vi "Host_HoppingScan(XY_FPGAWithin).vi"() -> ()   [LabVIEW 2014]
uses:
  <vilib>/userdefined/High Color/nirio_resource_hc.ctl
  <vilib>/Math Plots/3D Math Plots/3D Surface/3D Surface XCtrl/3D Surface.xctl
  <vilib>/FPGAPlugInAG/PCIe-7851R/niLvFpga_Open_PCIe-7851R.vi
  <vilib>/rvi/interface/common/dynamic/niFpgaDynamicAddResources.vi
  <vilib>/Utility/error.llb/Error Cluster From Error Code.vi
  <vilib>/rvi/errors/niLvFpgaAdjustHostInterfaceError.vi
  <vilib>/FPGAPlugInAG/Dynamic/niLvFpga_Run_Dynamic.vi
  <vilib>/FPGAPlugInAG/Dynamic/niLvFpga_Close_Dynamic.vi
  <vilib>/Math Plots/3D Math Plots/3D Surface/3D Surface Datatype/Public/Plot Helper (Matrix).vi
  <vilib>/rvi/interface/nirviOpenFPGA/nirviOpenFPGA.xnode
  FPGA Bitfiles/XZFPGAWithinHopp_FPGATarget_HoppingStepModif_nhH-EM1Hrjw.lvbitx
  <vilib>/rvi/interface/nirviReadWriteControl/nirviReadWriteControl.xnode
  <vilib>/rvi/interface/nirviMethod/nirviMethod.xnode
  <vilib>/rvi/interface/nirviCloseFPGA/nirviCloseFPGA.xnode
  NiFpgaLv.dll
  <vilib>/rvi/interface/Simulation/niFpgaSimulationCallBeginRW.vi
  <vilib>/FPGAPlugInAG/Dynamic/niLvFpga_ReadFifo_Dynamic.vi
  <vilib>/rvi/errors/niLvFpgaMergeErrorWithErrorCode.vi
  <vilib>/Math Plots/3D Math Plots/3D Surface/3D Surface Datatype/3D Surface Datatype.lvclass
panel:
  out "YGets":i32
  out "XGets":u32
  out "ZPos":i16(graph)
  out "3D Surface":refnum<class "3D Plot Datatype.lvclass">[](xcontrol)
  in  "stop":bool
  in  "PIXYZ":T1
  in  "InitZOffset":i32
  in  "MajorWithdraw":i32
  in  "YInitPos um":dbl
  in  "YStepLen um":dbl
  in  "YNum":i32
  in  "XInitPos um":dbl
  in  "XStepLen um":dbl
  in  "XNum":i32
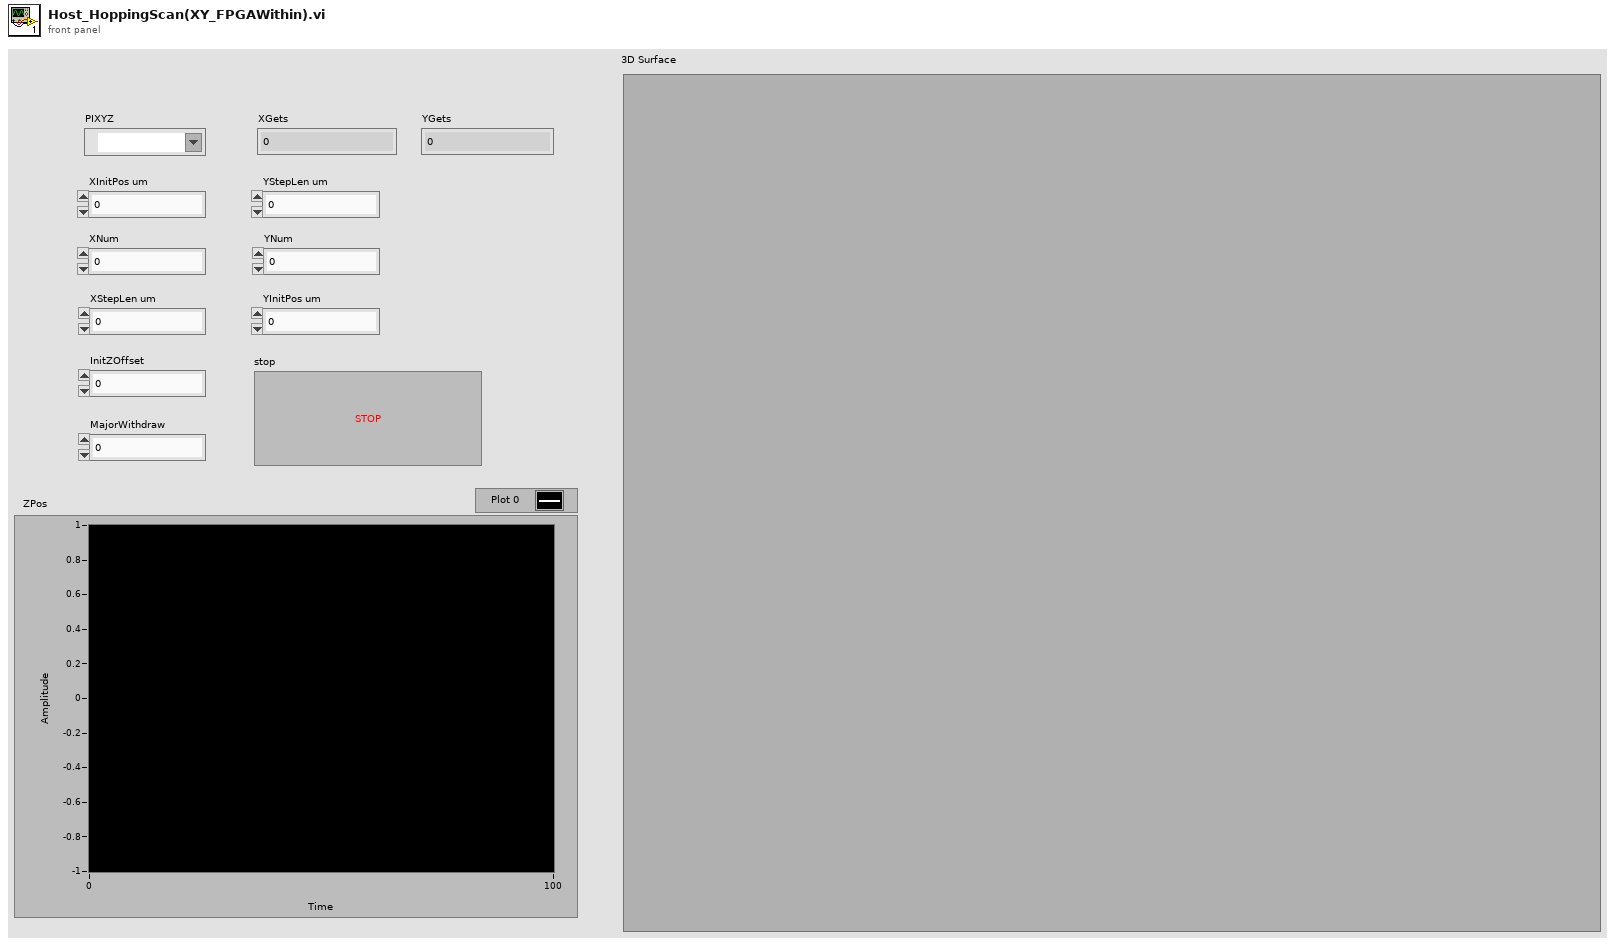
[diagram p1: front panel]
types:
  T1 = typedef "nirio_resource_hc.ctl" = tag
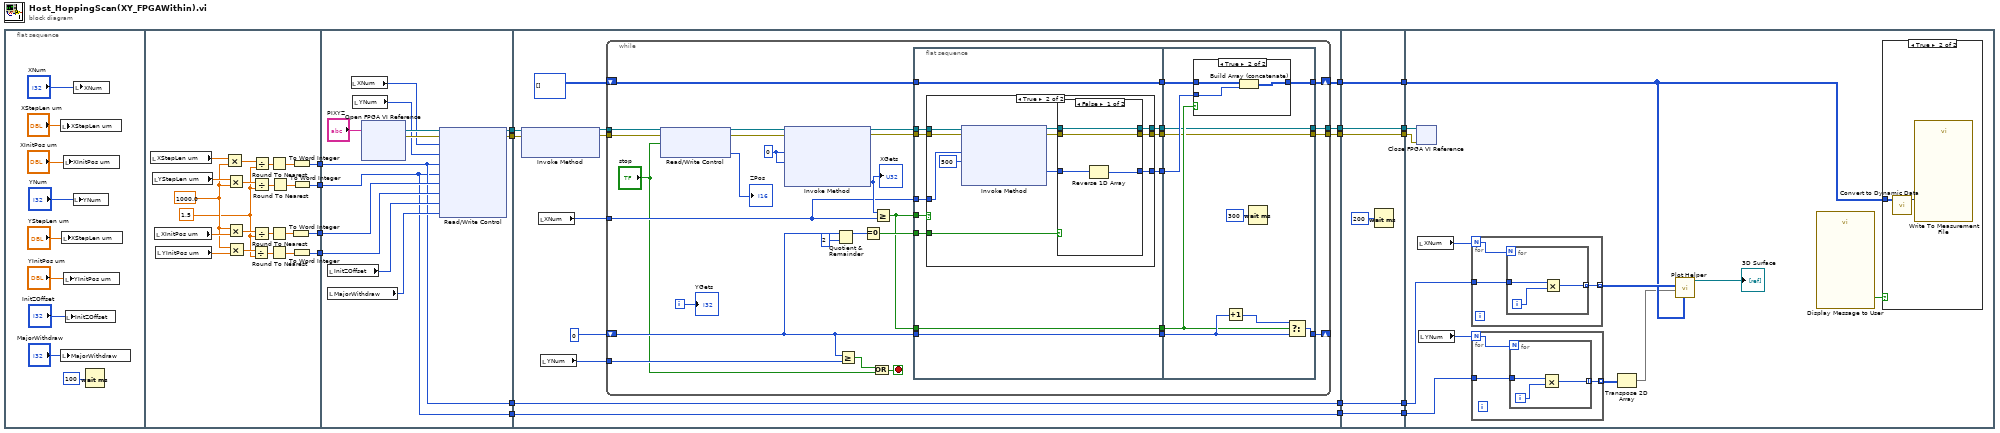
[diagram p0: block diagram]
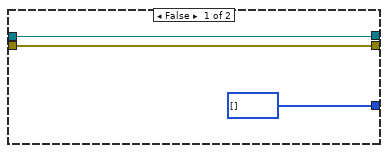
[diagram p2: hidden frame]
diagram:
  n1 = flat-sequence {
    tunnel: [w41] -> w16
    tunnel: [w40] -> w15
    tunnel: [w29] -> w14
    tunnel: [w28] -> w13
    tunnel: [w59] -> w18
    tunnel: [w58] -> w17
    tunnel: w16 -> [w51]
    tunnel: w15 -> [w50]
    tunnel: w14 -> [w55]
    tunnel: w13 -> [w54]
    tunnel: [w51] -> w6
    tunnel: [w50] -> w4
    tunnel: w18 -> [w75]
    tunnel: w17 -> [w74]
    tunnel: [w67] -> w11
    tunnel: [w66] -> w10
    tunnel: [w65] -> w9
    tunnel: w6 -> [w63]
    tunnel: [w64] -> w5
    tunnel: w4 -> [w64]
    tunnel: [w63] -> w3
    tunnel: [w157] -> w12
    tunnel: w11 -> [w157]
    tunnel: w10 -> [w156]
    tunnel: w9 -> [w155]
    tunnel: [w156] -> w8
    tunnel: [w155] -> w7
    tunnel: w5 -> [w153]
    tunnel: w3 -> [w154]
    tunnel: [w154] -> w2
    tunnel: [w153] -> w1
    tunnel: w12 -> [w161]
    tunnel: w8 -> [w170]
    tunnel: w7 -> [w169]
    tunnel: w2 -> [w165]
    tunnel: w1 -> [w164]
    frame #0 {
      n2 = local write "XStepLen um"("XStepLen um") -> ()
      n3 = local write "MajorWithdraw"("MajorWithdraw") -> ()
      n4 = local write "XStepLen um"("YStepLen um") -> ()
      n5 = local write "XInitPos um"("XInitPos um") -> ()
      n6 = local write "YInitPos um"("YInitPos um") -> ()
      n7 = local write "InitZOffset"("InitZOffset") -> ()
      n8 = local write "YNum"("YNum") -> ()
      n9 = local write "XNum"("XNum") -> ()
      n10 = Wait (ms)(milliseconds to wait=u32 100) -> ()  [unwired: 1 out]
    }
    frame #1 {
      w30 = 1.5
      w37 = 1000.0
      n11 = local read "XStepLen um"() -> (w47:dbl)
      n12 = local read "YStepLen um"() -> (w46:dbl)
      n13 = local read "XInitPos um"() -> (w39:dbl)
      n14 = local read "YInitPos um"() -> (w38:dbl)
      n15 = Multiply(x=w47, y=w37) -> (x*y=w48:dbl)
      n16 = Multiply(x=w46, y=w37) -> (x*y=w49:dbl)
      n17 = Multiply(x=w37, y=w39) -> (x*y=w32:dbl)
      n18 = Multiply(x=w37, y=w38) -> (x*y=w31:dbl)
      n19 = Divide(x=w31, y=w30) -> (x/y=w35:dbl)
      n20 = Divide(x=w49, y=w30) -> (x/y=w44:dbl)
      n21 = Divide(x=w32, y=w30) -> (x/y=w36:dbl)
      n22 = Divide(x=w48, y=w30) -> (x/y=w45:dbl)
      n23 = Round To Nearest(number=w36) -> (nearest integer value=w34:dbl)
      n24 = Round To Nearest(number=w45) -> (nearest integer value=w43:dbl)
      n25 = Round To Nearest(number=w35) -> (nearest integer value=w33:dbl)
      n26 = Round To Nearest(number=w44) -> (nearest integer value=w42:dbl)
      n27 = To Word Integer(number=w34) -> (16bit integer=w29:i16)
      n28 = To Word Integer(number=w43) -> (16bit integer=w41:i16)
      n29 = To Word Integer(number=w33) -> (16bit integer=w28:i16)
      n30 = To Word Integer(number=w42) -> (16bit integer=w40:i16)
    }
    frame #2 {
      n31 = local read "InitZOffset"() -> (w53:i32)
      n32 = local read "MajorWithdraw"() -> (w52:i32)
      n33 = local read "XNum"() -> (w57:i32)
      n34 = local read "YNum"() -> (w56:i32)
      n35 = xnode "Open FPGA VI Reference"("resource name"="PIXYZ") -> ("FPGA VI Reference Out"=w61:refnum<k20>, "error out"=w60:errorcluster)  [unwired: 1 in]
      n36 = xnode "Read/Write Control"("FPGA VI Reference In"=w61, "error in"=w60, "XNum"=w57, "YNum"=w56, "XStepIndex"=w51, "YStepIndex"=w50, "XOffset"=w55, "YOffset"=w54, "ZOffset"=w53, "MajorWithdraw"=w52) -> ("FPGA VI Reference Out"=w59:refnum<k20>, "error out"=w58:errorcluster)
    }
    frame #3 {
      n37 = xnode "Invoke Method"("FPGA VI Reference In"=w75, "error in"=w74) -> ("FPGA VI Reference Out"=w73:refnum<k20>, "error out"=w72:errorcluster)  [unwired: 1 in]
      n38 = local read "XNum"() -> (w70:i32)
      n39 = local read "YNum"() -> (w69:i32)
      n40 = while {
        tunnel: w73 -> [w84]
        tunnel: w72 -> [w83]
        tunnel: w70 -> [w102]
        tunnel: w69 -> [w101]
        shift-right: [w91] -> _
        shift-left: 0 -> [w100]
        shift-right: [w88] -> w67
        shift-left: i16[][] [] -> [w90]
        tunnel: [w86] -> w66
        tunnel: [w85] -> w65
        i -> [w76]
        stop <- w80 stop-if-true
        w106 = 0
        n41 = xnode "Read/Write Control"("FPGA VI Reference In"=w84, "error in"=w83, "stop"="stop") -> ("FPGA VI Reference Out"=w82:refnum<k20>, "error out"=w81:errorcluster, "Waveform Chart"=→"ZPos":i16)
        n42 = xnode "Invoke Method"("FPGA VI Reference In"=w82, "error in"=w81, "Number of Elements"=w106, "Timeout (ms)"=w106) -> ("FPGA VI Reference Out"=w104:refnum<k20>, "error out"=w103:errorcluster, "Elements Remaining"=w105:u32)  [unwired: 1 out]
        "XGets" <- w105
        n43 = Quotient & Remainder(x=w100, y=2) -> (x-y*floor(x/y)=w98:i32)  [unwired: 1 out]
        n44 = Greater Or Equal?(x=w100, y=w101) -> (x >= y?=w79:bool)
        n45 = Equal To 0?(x=w98) -> (x = 0?=w97:bool)
        n46 = Or(x=w79, y="stop") -> (x .or. y?=w80:bool)
        n47 = Greater Or Equal?(x=w105, y=w102) -> (x >= y?=w92:bool)
        n48 = flat-sequence {
          tunnel: w104 -> [w117]
          tunnel: w103 -> [w116]
          tunnel: w92 -> [w115]
          tunnel: w102 -> [w114]
          tunnel: w100 -> [w113]
          tunnel: w97 -> [w112]
          tunnel: [w113] -> w96
          tunnel: [w111] -> w95
          tunnel: [w110] -> w94
          tunnel: [w109] -> w93
          tunnel: w92 -> [w109]
          tunnel: w90 -> [w108]
          tunnel: [w108] -> w89
          tunnel: [w107] -> w87
          tunnel: w96 -> [w148]
          tunnel: w95 -> [w141]
          tunnel: w94 -> [w140]
          tunnel: w93 -> [w143]
          tunnel: [w146] -> w91
          tunnel: w89 -> [w145]
          tunnel: [w144] -> w88
          tunnel: w87 -> [w142]
          tunnel: [w141] -> w86
          tunnel: [w140] -> w85
          frame #0 {
            n49 = case shown="True" w115 {
              tunnel: w117 -> [w120 w131]
              tunnel: w116 -> [w119 w130]
              tunnel: w114 -> [_ w129]
              tunnel: w112 -> [_ w127]
              tunnel: [w120 w126] -> w111
              tunnel: [w119 w123] -> w110
              tunnel: [i16[] [] ("Data") w121] -> w107
              frame False {
              }
              frame True {
                n50 = xnode "Invoke Method"("FPGA VI Reference In"=w131, "error in"=w130, "Number of Elements"=w129, "Timeout (ms)"=500) -> ("FPGA VI Reference Out"=w125:refnum<k20>, "error out"=w124:errorcluster, "Data"=w122:i16[])  [unwired: 1 out]
                n51 = case shown="False" w127 {
                  tunnel: [w135 w138] -> w126
                  tunnel: w125 -> [w135 w138]
                  tunnel: w124 -> [w134 w137]
                  tunnel: [w134 w137] -> w123
                  tunnel: w122 -> [w133 w136]
                  tunnel: [w132 w136] -> w121
                  frame False {
                    n52 = Reverse 1D Array(array=w133) -> (reversed array=w132:i16[])
                  }
                  frame True {
                  }
                }
              }
            }
          }
          frame #1 {
            n53 = case shown="True" w143 {
              tunnel: w145 -> [w149 w152]
              tunnel: [w149 w151] -> w144
              tunnel: w142 -> [_ w150]
              frame False {
              }
              frame True {
                n54 = Build Array (concatenate)(w152, w150) -> (w151:i16[][])
              }
            }
            n55 = Increment(x=w148) -> (x+1=w147:i32)
            n56 = Wait (ms)(milliseconds to wait=u32 300) -> ()  [unwired: 1 out]
            n57 = Select(t=w147, s=w143, f=w148) -> (s? t:f=w146:i32)
          }
        }
        "YGets" <- w76
      }
    }
    frame #4 {
      n58 = Wait (ms)(milliseconds to wait=u32 200) -> ()  [unwired: 1 out]
    }
    frame #5 {
      n59 = xnode "Close FPGA VI Reference"("FPGA VI Reference In"=w170, "error in"=w169) -> ()  [unwired: 1 out]
      n60 = local read "XNum"() -> (w167:i32)
      n61 = local read "YNum"() -> (w166:i32)
      n62 = for {
        N: w167 -> [w177]
        tunnel: w165 -> [w179]
        tunnel: [w178] -> w162 mode=indexing
        n63 = for {
          N: w177 -> [_]
          tunnel: w179 -> [w182]
          tunnel: [w180] -> w178 mode=indexing
          i -> [w181]
          n64 = Multiply(x=w182, y=w181) -> (x*y=w180:i32)
        }
      }
      n65 = for {
        N: w166 -> [w171]
        tunnel: w164 -> [w173]
        tunnel: [w172] -> w160 mode=indexing
        n66 = for {
          N: w171 -> [_]
          tunnel: w173 -> [w176]
          tunnel: [w174] -> w172 mode=indexing
          i -> [w175]
          n67 = Multiply(x=w176, y=w175) -> (x*y=w174:i32)
        }
      }
      n68 = Transpose 2D Array(2D array=w160) -> (transposed array=w159:i32[][])
      n69 = call-poly <vilib>:"Plot Helper.vi"("z matrix"=w161, "y matrix"=w159, "x matrix"=w162) -> ("3D Plot lvclass Array out"=→"3D Surface":refnum<class "3D Plot Datatype.lvclass">[])  [unwired: 3 in, 5 out]
      n70 = call "Display Message to User"() -> ("OK"=w168:bool)  [unwired: 10 in, 1 out]
      n71 = case shown="True" w168 {
        tunnel: w161 -> [_ w184]
        frame False {
        }
        frame True {
          n72 = call "Convert to Dynamic Data"("2D Array"=w184) -> ("Dynamic Data Type"=w183:dynamicdata)  [unwired: 3 in]
          n73 = call "Write To Measurement File"("Signals"=w183) -> ()  [unwired: 16 in, 3 out]
        }
      }
    }
  }
